vi "Connect to Server.vi"(4 "timeout (1000 ms)":i32=1000, 5 "Connect Flags":T3, 6 "Keep Alive (s)":u16, 7 "Payload":T2, 8 "error in (no error)":errorcluster, 9 "remote port (8883)":u16=8883, 10 "address (localhost)":string="localhost", 11 "Client in":refnum<class "Client.lvclass">) -> (0 "error out":errorcluster, 1 "timed out":bool, 2 "Server Response":T1, 3 "Client out":refnum<class "Client.lvclass">)   [LabVIEW 2013, in "MQTT Server.lvlib" / "Client.lvclass"]
uses:
  Client.lvclass
  Control Packets/CONNECT/ConnectFlags -- cluster.ctl
  Control Packets/CONNACK/Connect Return Code -- enum.ctl
  Control Packets/CONNACK/CONNACK.lvclass
  Client.lvclass/Client.ctl
  Server/Connection/TCPConnection.lvclass
  Control Packets/CONNECT/CONNECT.lvclass
  Control Packets/ControlPacket/ControlPacket.lvclass
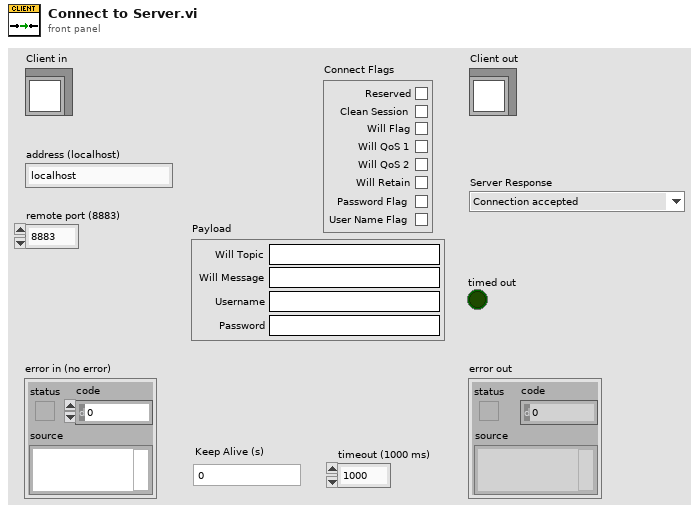
[diagram p1: front panel]
types:
  T1 = typedef "CONNACK.lvclass/Connect Return Code -- enum.ctl" = enum16{"Connection accepted", "Unacceptable protocol version", "Identifier Rejected", "Server Unavailable", "Bad Username or Password", "Not Authorized"}
  T2 = cluster{"Will Topic":string, "Will Message":string, "Username":string, "Password":string}
  T3 = typedef "CONNECT.lvclass/ConnectFlags -- cluster.ctl" = cluster{"Reserved":bool, "Clean Session":bool, "Will Flag":bool, "Will QoS 1":bool, "Will QoS 2":bool, "Will Retain":bool, "Password Flag":bool, "User Name Flag":bool}
  T4 = enum16{"Standard", "Buffered", "CRLF", "Immediate"}
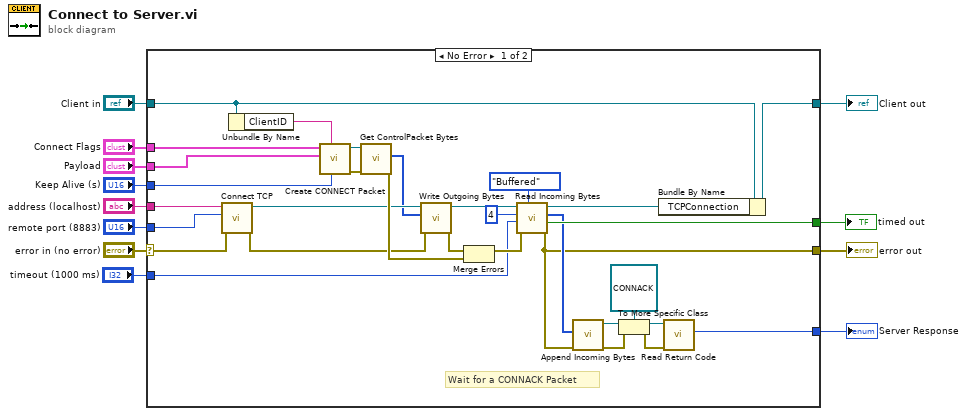
[diagram p0: block diagram]
diagram:
  n1 = case shown="No Error" "error in (no error)" {
    selector: "error in (no error)" -> [w40 w45]
    tunnel: [w14 w45] -> w11
    tunnel: [w43 w44] -> w9
    tunnel: "Client in" -> [w32 w44]
    tunnel: "address (localhost)" -> [w42 _]
    tunnel: "remote port (8883)" -> [w41 _]
    tunnel: "Connect Flags" -> [w36 _]
    tunnel: "Payload" -> [w35 _]
    tunnel: "Keep Alive (s)" -> [w33 _]
    tunnel: [w22 _] -> w3
    tunnel: "timeout (1000 ms)" -> [w21 _]
    tunnel: [w13 _] -> w1
    frame No Error {
      # "Wait for a CONNACK Packet"
      n2 = call "Connect TCP.vi"("error in (no error)"=w40, "remote port (80)"=w41, "address (localhost)"=w42) -> ("error out"=w30:errorcluster, "TCPConnection out"=w31:refnum<class "TCPConnection.lvclass">)  [unwired: 7 in]
      n3 = Unbundle By Name(w32) -> ("ClientID"=w37:string)
      n4 = call "Create CONNECT Packet.vi"("Keep Alive (s)"=w33, "Client ID (empty: generate new)"=w37, "Payload"=w35, "Connect Flags"=w36) -> ("error out"=w38:errorcluster, "CONNECT"=w39:refnum<class "CONNECT.lvclass">)  [unwired: 6 in]
      n5 = call "Get ControlPacket Bytes.vi"("error in (no error)"=w38, "ControlPacket"=w39) -> ("error out"=w34:errorcluster, "Bytes Stream"=w28:u8[])  [unwired: 7 in, 1 out]
      n6 = call "Write Outgoing Bytes.vi"("error in (no error)"=w30, "Bytes"=w28, "TCPConnection in"=w31) -> ("error out"=w29:errorcluster, "TCPConnection out"=w25:refnum<class "TCPConnection.lvclass">)  [unwired: 7 in]
      n7 = Merge Errors(w29, w34) -> (w23:errorcluster)
      n8 = call "Read Incoming Bytes.vi"("mode (standard)"=T4."Buffered", "error in (no error)"=w23, "timeout (1000 ms)"=w21, "bytes to read (100)"=4 ("bytes to read"), "TCPConnection in"=w25) -> ("error out"=w14:errorcluster, "timed out"=w22:bool, "Bytes"=w15:u8[], "TCPConnection out"=w24:refnum<class "TCPConnection.lvclass">)  [unwired: 3 in]
      n9 = call "Append Incoming Bytes.vi"("error in (no error)"=w14, "Incoming Packets"=w15) -> ("error out"=w16:errorcluster, "ControlPacket"=w20:refnum<class "ControlPacket.lvclass">)  [unwired: 6 in, 2 out]
      n10 = To More Specific Class(target class=refnum<class "CONNACK.lvclass"> refnum ("CONNACK.lvclass"), reference=w20, error in=w16) -> (specific class reference=w18:refnum<class "CONNACK.lvclass">, error out=w17:errorcluster)
      n11 = Bundle By Name(cluster=w32, "TCPConnection"=w24) -> (w43:refnum<class "Client.lvclass">)
      n12 = call "Read Return Code.vi"("error in (no error)"=w17, "CONNACK in"=w18) -> ("Return Code"=w13:T1)  [unwired: 7 in, 2 out]
    }
    frame Error {
    }
  }
  "error out" <- w11
  "Client out" <- w9
  "timed out" <- w3
  "Server Response" <- w1
